vi "混合模块站号转换.vi"(11 "Slave ID输入":T1) -> (3 "Slave ID输出":T1)   [LabVIEW 2016, in "质控单元V1.lvlib"]
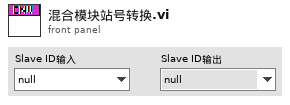
[diagram p1: front panel]
types:
  T1 = typedef "质控单元V1.lvlib/质控slave id.ctl" = enum16{"null", "氨氮", "总磷", "CODMn", "CODCr", "总氮"}
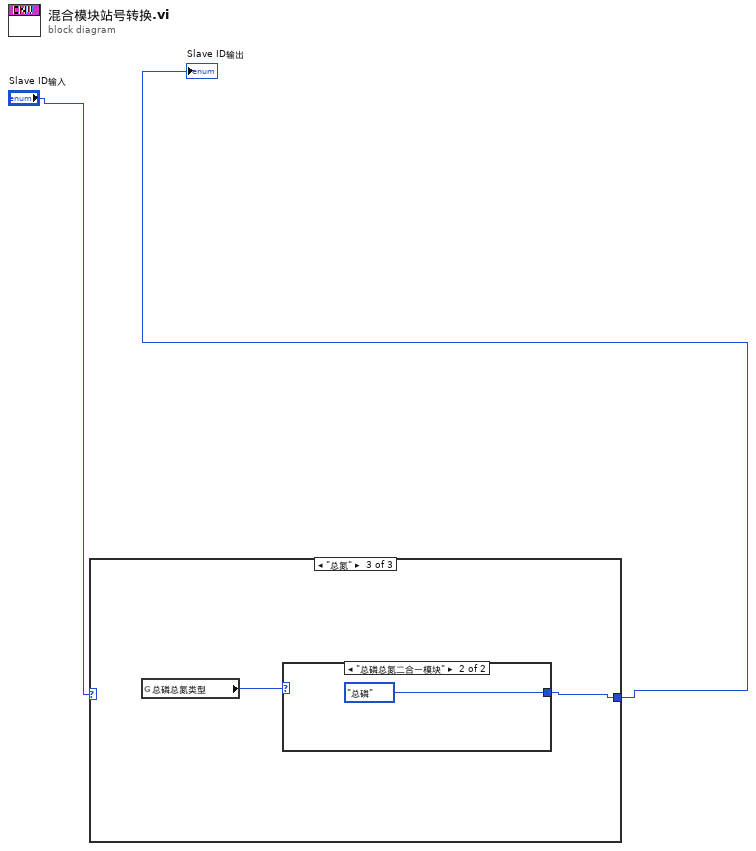
[diagram p0: block diagram]
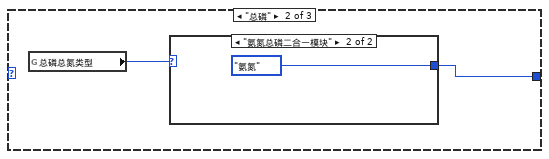
[diagram p3: hidden frame]
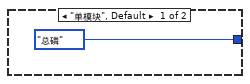
[diagram p4: hidden frame]
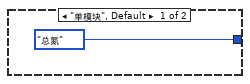
[diagram p5: hidden frame]
diagram:
  n1 = case shown="\"总氮\"" "Slave ID输入" {
    selector: "Slave ID输入" -> [w3 _ _]
    tunnel: [w3 w4 w8] -> w2
    frame "null", Default {
    }
    frame "总磷" {
      n2 = global read "系统交互.vi" "总磷总氮类型"() -> (w5:enum16{"单模块", "总磷总氮二合一模块", "氨氮总磷二合一模块"})
      n3 = case shown="\"氨氮总磷二合一模块\"" w5 {
        tunnel: [质控slave_id."总磷" ("Slave ID") 质控slave_id."氨氮" ("Slave ID")] -> w4
        frame "单模块", Default {
        }
        frame "氨氮总磷二合一模块" {
        }
      }
    }
    frame "总氮" {
      n4 = global read "系统交互.vi" "总磷总氮类型"() -> (w9:enum16{"单模块", "总磷总氮二合一模块", "氨氮总磷二合一模块"})
      n5 = case shown="\"总磷总氮二合一模块\"" w9 {
        tunnel: [质控slave_id."总氮" ("Slave ID") 质控slave_id."总磷" ("Slave ID")] -> w8
        frame "单模块", Default {
        }
        frame "总磷总氮二合一模块" {
        }
      }
    }
  }
  "Slave ID输出" <- w2
